vi "komutator.vi"(11 "Numeric":u8) -> ()   [LabVIEW 2018]
doc: "Ustawia komutator."
uses:
  Open_device_2017.llb/Select_Instr.ctl
panel:
  out "error out":errorcluster
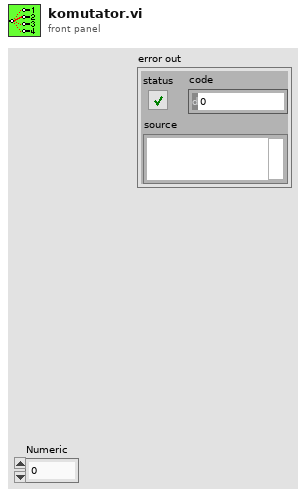
[diagram p1: front panel]
types:
  T1 = typedef "Select_Instr.ctl" = string
  T2 = cluster{"VISA resource name":refnum<visa-resource-name>}
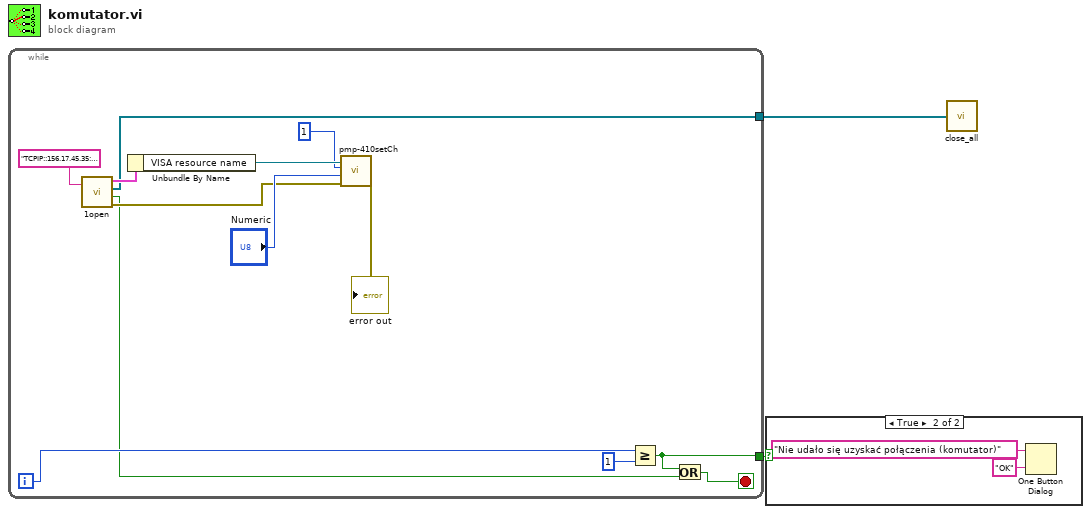
[diagram p0: block diagram]
diagram:
  n1 = while {
    tunnel: [w5] -> w2
    tunnel: [w3] -> w1
    i -> [w8]
    stop <- w4 stop-if-true
    n2 = call "1open.vi"("VISA resource name"=T1 "TCPIP::156.17.45.35::inst104::INSTR" ("Select_Instrument")) -> ("InstrCluster"=w14:T2, "InstrArray"=w5:refnum<visa-resource-name>[], "Open OK (true)"=w6:bool, "error out"=w9:errorcluster)  [unwired: 1 in]
    n3 = Unbundle By Name(w14) -> ("VISA resource name"=w13:refnum<visa-resource-name>)
    n4 = call "pmp-410setCh.vi"("error in (no error)"=w9, "Channel"="Numeric", "Slave#"=1, "VISA Refnum in"=w13) -> ("error out"=→"error out":errorcluster)  [unwired: 6 in, 1 out]
    n5 = Greater Or Equal?(x=w8, y=1) -> (x >= y?=w3:bool)
    n6 = Or(x=w3, y=w6) -> (x .or. y?=w4:bool)
  }
  n7 = case shown="True" w1 {
    frame False {
    }
    frame True {
      n8 = One Button Dialog(message="Nie udało się uzyskać połączenia (komutator)", button name ("OK")="OK") -> ()  [unwired: 1 out]
    }
  }
  n9 = call "close_all.vi"("OpenRes"=w2) -> ()  [unwired: 1 out]
